vi "Read timeout.vi"(8 "error in (no error)":errorcluster, 11 "Test Suite in":refnum<class "Test Suite.lvclass">) -> (0 "error out":errorcluster, 2 "timeout":i32=1000, 3 "Test Suite out":refnum<class "Test Suite.lvclass">)   [LabVIEW 2013, in "Caraya.lvlib" / "Test Suite.lvclass"]
uses:
  Test Suite.lvclass
  Test Suite.lvclass/Test Suite.ctl
  Properties.Suite/Properties.Suite.lvclass/Properties.Suite.ctl
  Properties.Suite/Properties.Suite.lvclass
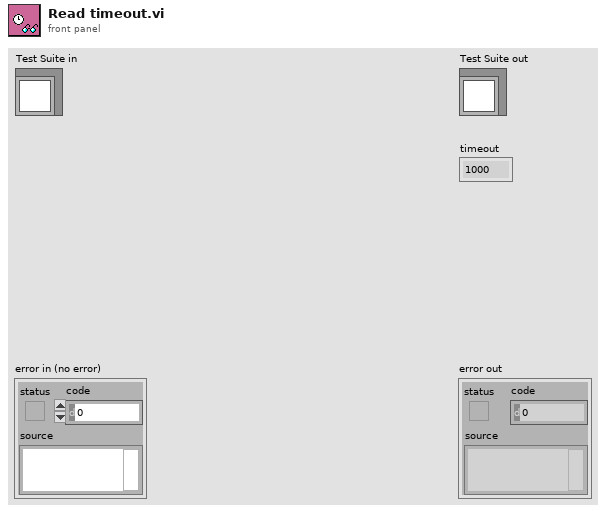
[diagram p1: front panel]
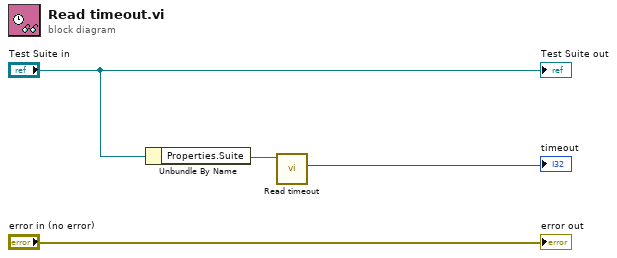
[diagram p0: block diagram]
diagram:
  n1 = Unbundle By Name("Test Suite in") -> ("Properties.Suite"=w2:refnum<class "Properties.Suite.lvclass">)
  n2 = call "Read timeout.vi"("Properties.Suite in"=w2) -> ("timeout"=→"timeout":i32)  [unwired: 9 in, 1 out]
  "error out" <- "error in (no error)"
  "Test Suite out" <- "Test Suite in"
